vi "Get Graphic Control Extension.vi"(8 "error in (no error)":errorcluster caption="错误输入（无错误）", 11 "Gif Image 输入":refnum<class "Gif Image.lvclass"> caption="DNL_LabVIEW Object in") -> (0 "error out":errorcluster caption="错误输出", 1 "Graphic Control ExtPacked Field":T1, 2 "Graphic Control Extension":T2 {"Graphic Control Label(1)" format="0x%02x" items=["Image Seperator"=44, "Extension Introducer"=33, "Graphic Control Label"=249, "Comment Label"=254, "PlainText Label"=1, "Gif Trailor"=59, "Application Label"=255]; "ID(1)" format="0x%02x" items=["Image Seperator"=44, "Extension Introducer"=33, "Graphic Control Label"=249, "Comment Label"=254, "PlainText Label"=1, "Gif Trailor"=59, "Application Label"=255]}, 3 "Gif Image 输出":refnum<class "Gif Image.lvclass"> caption="DNL_LabVIEW Object out")   [LabVIEW 2012, in "Picture Box Tools.lvlib" / "Gif Image.lvclass"]
uses:
  Gif Image.lvclass
  Control/Graphic Control Extension.ctl
  Control/ID Charactor.ctl
  Control/Graphic Control ExtPackedField.ctl
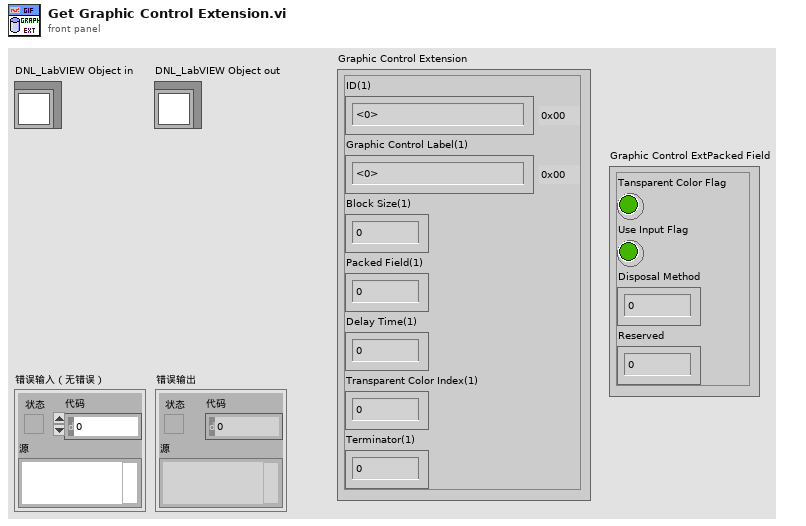
[diagram p1: front panel]
types:
  T1 = typedef "Picture Box Tools.lvlib/Gif Image.lvclass/Graphic Control ExtPackedField.ctl" = cluster{"Tansparent Color Flag":bool, "Use Input Flag":bool, "Disposal Method":u8, "Reserved":u8}
  T2 = typedef "Picture Box Tools.lvlib/Gif Image.lvclass/Graphic Control Extension.ctl" = cluster{"ID(1)":T3, "Graphic Control Label(1)":T3, "Block Size(1)":i8, "Packed Field(1)":u8, "Delay Time(1)":u8, "Transparent Color Index(1)":u8, "Terminator(1)":dbl}
  T3 = typedef "Picture Box Tools.lvlib/Gif Image.lvclass/ID Charactor.ctl" = u8
  T4 = enum16{"big-endian, network order", "native, host order", "little-endian"}
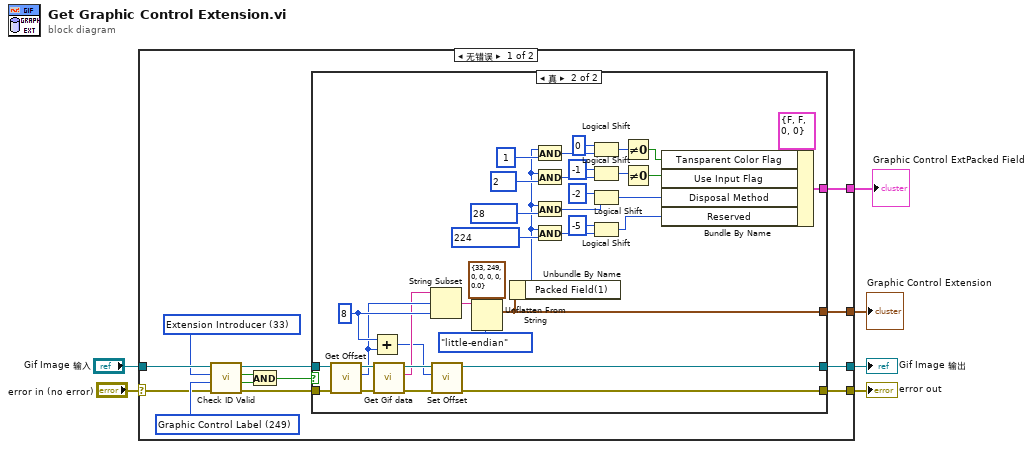
[diagram p0: block diagram]
diagram:
  n1 = case shown="无错误" "error in (no error)" {
    selector: "error in (no error)" -> [w12 w60]
    tunnel: [w10 w60] -> w5
    tunnel: "Gif Image 输入" -> [w19 w59]
    tunnel: [w9 w59] -> w3
    tunnel: [w8 _] -> w2
    tunnel: [w7 _] -> w1
    frame No Error {
      w17 = T3 249 items=["Image Seperator"=44, "Extension Introducer"=33, "Graphic Control Label"=249, "Comment Label"=254, "PlainText Label"=1, "Gif Trailor"=59, "Application Label"=255] ("Label")
      w18 = T3 33 items=["Image Seperator"=44, "Extension Introducer"=33, "Graphic Control Label"=249, "Comment Label"=254, "PlainText Label"=1, "Gif Trailor"=59, "Application Label"=255] ("ID")
      n2 = call "Check ID Valid.vi"("error in (no error)"=w12, "Label"=w17, "ID"=w18, "Gif Image 输入"=w19) -> ("error out"=w11:errorcluster, "Label Valid"=w15:bool, "ID Valid"=w16:bool, "Gif Image 输出"=w13:refnum<class "Gif Image.lvclass">)  [unwired: 4 in]
      n3 = And(x=w16, y=w15) -> (x .and. y?=w14:bool)
      n4 = case shown="真" w14 {
        tunnel: w13 -> [w20 w58]
        tunnel: w11 -> [w21 w57]
        tunnel: [w21 w53] -> w10
        tunnel: [w20 w52] -> w9
        tunnel: [_ w43] -> w8
        tunnel: [_ w28] -> w7
        frame False {
        }
        frame True {
          w50 = 8 ("长度（剩余）")
          n5 = call "Get Offset.vi"("error in (no error)"=w57, "Gif Image输入"=w58) -> ("error out"=w56:errorcluster, "Offset"=w49:i32, "Gif Image输出"=w55:refnum<class "Gif Image.lvclass">)  [unwired: 7 in]
          n6 = Add(x=w50, y=w49) -> (x+y=w47:i32)
          n7 = call "Get Gif data.vi"("error in (no error)"=w56, "Gif Image输入"=w55) -> ("error out"=w51:errorcluster, "Gif data"=w48:string, "Gif Image输出"=w54:refnum<class "Gif Image.lvclass">)  [unwired: 7 in]
          n8 = String Subset(string=w48, offset (0)=w49, length (rest)=w50) -> (substring=w46:string)
          n9 = call "Set Offset.vi"("error in (no error)"=w51, "Offset"=w47, "Gif Image输入"=w54) -> ("error out"=w53:errorcluster, "Gif Image输出"=w52:refnum<class "Gif Image.lvclass">)  [unwired: 7 in]
          n10 = Unflatten From String(type=T2 {"ID(1)"=33, "Graphic Control Label(1)"=249, "Block Size(1)"=0, "Packed Field(1)"=0, "Delay Time(1)"=0, "Transparent Color Index(1)"=0, "Terminator(1)"=0.0} ("Graphic Control Extension"), binary string=w46, byte order (0:big-endian, network order)=T4."little-endian" ("字节顺序(0:big-endian, network order)")) -> (value=w43:T2)  [unwired: 2 in, 2 out]
          n11 = Unbundle By Name(w43) -> ("Packed Field(1)"=w30:u8)
          n12 = And(x=w30, y=u8 1 ("length (rest)")) -> (x .and. y?=w36:u8)
          n13 = And(x=w30, y=u8 2 ("length (rest)")) -> (x .and. y?=w37:u8)
          n14 = And(x=w30, y=u8 28 ("length (rest)")) -> (x .and. y?=w38:u8)
          n15 = And(x=w30, y=u8 224 ("length (rest)")) -> (x .and. y?=w35:u8)
          n16 = Logical Shift(y=0, x=w36) -> (x << y=w27:u8)
          n17 = Logical Shift(y=-1, x=w37) -> (x << y=w25:u8)
          n18 = Logical Shift(y=-2, x=w38) -> (x << y=w22:u8)
          n19 = Logical Shift(y=-5, x=w35) -> (x << y=w23:u8)
          n20 = Not Equal To 0?(x=w27) -> (x != 0?=w26:bool)
          n21 = Not Equal To 0?(x=w25) -> (x != 0?=w24:bool)
          n22 = Bundle By Name(cluster=T1 {"Tansparent Color Flag"=FALSE, "Use Input Flag"=FALSE, "Disposal Method"=0, "Reserved"=0} ("Graphic Control ExtPacked Field"), "Tansparent Color Flag"=w26, "Use Input Flag"=w24, "Disposal Method"=w22, "Reserved"=w23) -> (w28:T1)
        }
      }
    }
    frame Error {
    }
  }
  "error out" <- w5
  "Gif Image 输出" <- w3
  "Graphic Control ExtPacked Field" <- w1
  "Graphic Control Extension" <- w2
